vi "DAQmx立即写数字端口设置.vi"(8 "error in":errorcluster) -> (0 "error out":errorcluster, 3 "task out":refnum<k21>)   [LabVIEW 2010]
doc: "This VI configures a task.\n\nYour program typically should execute this configuration code only once. To use this code in a loop, use the DAQmx ClearTask VI in the same loop."
uses:
  <vilib>/DAQmx/create/channels.llb/DAQmx Create Channel (DO-Digital Output).vi
  C:/Program Files/National Instruments/LabVIEW 2010/resource/objmgr/daqmx.rc
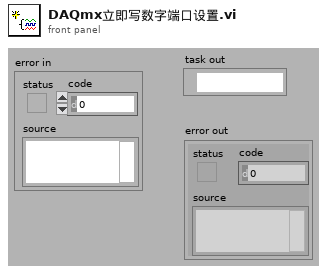
[diagram p1: front panel]
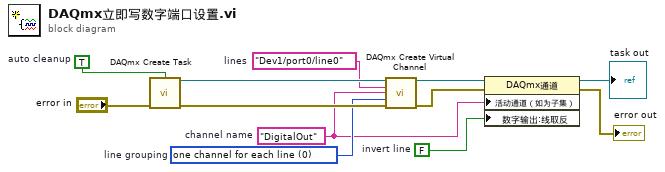
[diagram p0: block diagram]
diagram:
  w2 = FALSE  # invert line
  w7 = 0 items=["one channel for each line", "one channel for all lines"]  # line grouping
  w1 = "DigitalOut"  # channel name
  w8 = "Dev1/port0/line0"  # lines
  w9 = TRUE  # auto cleanup
  n1 = call <vilib>:"DAQmx Create Task.vi"("auto cleanup"=w9, "error in"="error in") -> ("task out"=w10:refnum<k21>, "error out"=w11:errorcluster)  [unwired: 12 in]
  n2 = call-poly <vilib>:"DAQmx Create Virtual Channel.vi"("task in"=w10, "lines"=w8, "name to assign"=w1, "line grouping"=w7, "error in"=w11) -> ("task out"=w6:refnum<k21>, "error out"=w5:errorcluster)  [unwired: 9 in]
  n3 = property class="DAQmx通道"(reference=w6, error in=w5, "活动通道（如为子集）"=w1, "数字输出:线取反"=w2) -> (reference out=→"task out":refnum<k21>, error out=→"error out":errorcluster)
